vi "Status Register.vi"(8 "error in (no error)":errorcluster, 9 "Register Bit(0)":i32 min=0 max=255 step=1, 10 "Status Register(0:Quest Event Enable Register)":u16(ring) items=["Quest Event Enable Register", "Quest Event Enable Register?", "Quest Event Register?", "Quest Enable Register (INST)", "Quest Enable Register? (INST)", "Quest Event Register? (INST)", "Operation Event Enable Register", "Operation Event Enable Register?", "Operation Event Register?", "Operation Enable Register (INST)", "Operation Enable Register? (INST)", "Operation Event Register? (INST)"], 11 "VISA resource name":refnum<visa-resource-name>) -> (0 "error out":errorcluster, 2 "Status Register Response":string, 3 "VISA resource name out":refnum<visa-resource-name>)   [LabVIEW 2018, in "Keithley KE22xx Series.lvlib"]
doc: "Sends query to the power supply and obtains the response from the instrument and sets particular bit of the specified register to 1."
uses:
  Keithley KE22xx Series.lvlib
panel:
  # "© 2012 Keithley Instruments, Inc. ALL RIGHTS RESERVED"
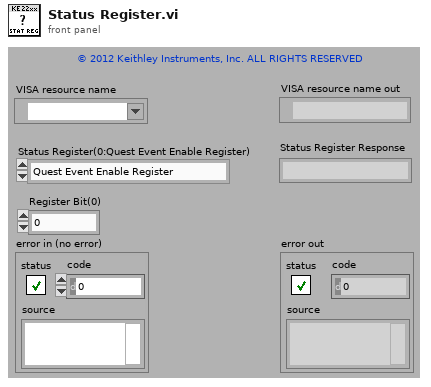
[diagram p1: front panel]
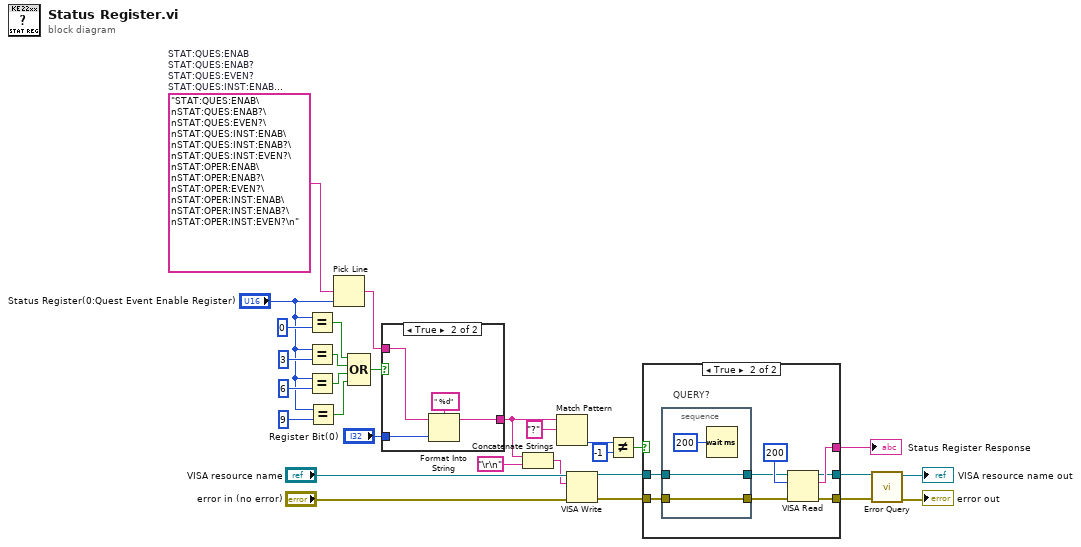
[diagram p0: block diagram]
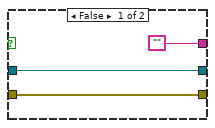
[diagram p2: hidden frame]
diagram:
  w27 = "STAT:QUES:ENAB\nSTAT:QUES:ENAB?\nSTAT:QUES:EVEN?\nSTAT:QUES:INST:ENAB\nSTAT:QUES:INST:ENAB?\nSTAT:QUES:INST:EVEN?\nSTAT:OPER:ENAB\nSTAT:OPER:ENAB?\nSTAT:OPER:EVEN?\nSTAT:OPER:INST:ENAB\nSTAT:OPER:INST:ENAB?\nSTAT:OPER:INST:EVEN?\n"  # STAT:QUES:ENAB STAT:QUES:ENAB? STAT:QUES:EVEN? STAT:QUES:INST:ENAB STAT:QUES:INST:ENAB? STAT:QUES:INST:EVEN? STAT:OPER:ENAB STAT:OPER:ENAB? STAT:OPER:EVEN? STAT:OPER:INST:ENAB STAT:OPER:INST:ENAB? STAT:OPER:INST:EVEN?
  n1 = Equal?(x="Status Register(0:Quest Event Enable Register)", y=u16 0) -> (x = y?=w5:bool)
  n2 = Equal?(x="Status Register(0:Quest Event Enable Register)", y=u16 3) -> (x = y?=w4:bool)
  n3 = Equal?(x="Status Register(0:Quest Event Enable Register)", y=u16 6) -> (x = y?=w3:bool)
  n4 = Equal?(x="Status Register(0:Quest Event Enable Register)", y=u16 9) -> (x = y?=w2:bool)
  n5 = Pick Line(multi-line string=w27, line index="Status Register(0:Quest Event Enable Register)") -> (output string=w23:string)  [unwired: 1 out]
  n6 = Compound Arithmetic op=OR(w5, w4, w3, w2) -> (w1:bool)
  n7 = case shown="True" w1 {
    tunnel: [w30 w33] -> w15
    tunnel: "Register Bit(0)" -> [_ w32]
    tunnel: w23 -> [w30 w31]
    frame False {
    }
    frame True {
      n8 = Format Into String(format string=" %d", initial string=w31, w32) -> (resulting string=w33:string)  [unwired: 1 in, 1 out]
    }
  }
  n9 = Concatenate Strings(w15, "\r\n") -> (w20:string)
  n10 = Match Pattern(string=w15, regular expression="?") -> (offset past match=w17:i32)  [unwired: 4 out]
  n11 = VISA Write(VISA resource name="VISA resource name", write buffer=w20, error in (no error)="error in (no error)") -> (VISA resource name out=w22:refnum<visa-resource-name>, error out=w21:errorcluster)  [unwired: 1 out]
  n12 = Not Equal?(x=w17, y=-1) -> (x != y?=w14:bool)
  n13 = case shown="True" w14 {
    tunnel: w22 -> [w36 w44]
    tunnel: w21 -> [w35 w43]
    tunnel: ["" ("read buffer") w40] -> w13
    tunnel: [w36 w39] -> w12
    tunnel: [w35 w38] -> w11
    frame False {
    }
    frame True {
      # "QUERY?"
      n14 = stacked-sequence {
        tunnel: w44 -> [w47]
        tunnel: w43 -> [w46]
        tunnel: [w47] -> w42
        tunnel: [w46] -> w41
        frame #0 {
          n15 = Wait (ms)(milliseconds to wait=u32 200) -> ()  [unwired: 1 out]
        }
      }
      n16 = VISA Read(VISA resource name=w42, byte count=u32 200, error in (no error)=w41) -> (VISA resource name out=w39:refnum<visa-resource-name>, read buffer=w40:string, error out=w38:errorcluster)  [unwired: 1 out]
    }
  }
  "Status Register Response" <- w13
  n17 = call "Error Query.vi"("error in (no error)"=w11, "VISA resource name"=w12) -> ("error out"=→"error out":errorcluster, "VISA resource name out"=→"VISA resource name out":refnum<visa-resource-name>)  [unwired: 6 in, 2 out]
